vi "WaitForArmError.vi"(8 "error in":errorcluster, 9 "Timeout (ms)":dbl, 10 "AllowedError":dbl) -> (0 "error out":errorcluster)   [LabVIEW 2015]
uses:
  MotorPositionGlobals.vi
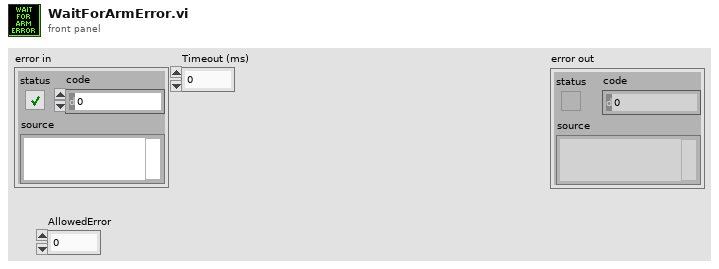
[diagram p1: front panel]
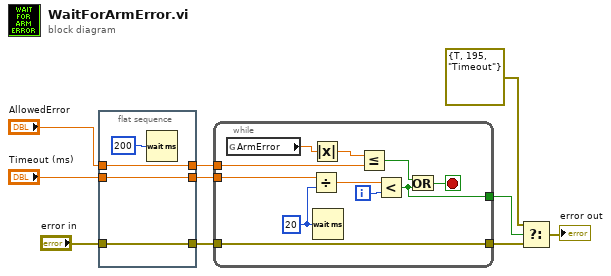
[diagram p0: block diagram]
diagram:
  n1 = flat-sequence {
    tunnel: "AllowedError" -> [w14]
    tunnel: [w14] -> w5
    tunnel: "Timeout (ms)" -> [w13]
    tunnel: [w13] -> w3
    tunnel: "error in" -> [w12]
    tunnel: [w12] -> w1
    frame #0 {
      n2 = Wait (ms)(milliseconds to wait=u32 200) -> ()  [unwired: 1 out]
    }
  }
  n3 = while {
    tunnel: w5 -> [w24]
    tunnel: w3 -> [w22]
    tunnel: [w17] -> w10
    tunnel: w1 -> [w16]
    tunnel: [w16] -> w7
    i -> [w18]
    stop <- w20 stop-if-true
    w21 = u32 20 ("milliseconds to wait")
    n4 = global read "MotorPositionGlobals.vi" "ArmError"() -> (w15:dbl)
    n5 = Divide(x=w22, y=w21) -> (x/y=w19:dbl)
    n6 = Absolute Value(x=w15) -> (abs(x)=w25:dbl)
    n7 = Wait (ms)(milliseconds to wait=w21) -> ()  [unwired: 1 out]
    n8 = Less Or Equal?(x=w25, y=w24) -> (x <= y?=w23:bool)
    n9 = Less?(x=w19, y=w18) -> (x < y?=w17:bool)
    n10 = Or(x=w23, y=w17) -> (x .or. y?=w20:bool)
  }
  n11 = Select(t=errorcluster {"status"=TRUE, "code"=195, "source"="Timeout"}, s=w10, f=w7) -> (s? t:f=→"error out":errorcluster)
